vi "Fetch Waveform Measurement In Memory.vi"(6 "Measurement Number (0: Measurement 1)":i32(ring) items=["Measurement 1", "Measurement 2", "Measurement 3", "Measurement 4"], 7 "Destination Channel (1: Channel 2)":u16(ring)=1 items=["Channel 1", "Channel 2", "Channel 3", "Channel 4", "Math", "D0", "D1", "D2", "D3", "D4", "D5", "D6", "D7", "D8", "D9", "D10", "D11", "D12", "D13", "D14", "D15", "Reference 1", "Reference 2", "Reference 3", "Reference 4", "Amplitude", "Frequency", "Phase"], 8 "error in (no error)":errorcluster, 9 "Measurement Function (21: Period)":i32(ring)=21 items=["Amplitude", "Area", "Burst Width", "Cycle Area", "Voltage Mean (cycle)", "Voltage RMS (cycle)", "Delay", "Fall Time", "Frequency", "Voltage High", "Voltage Low", "Voltage Max", "Voltage Mean", "Voltage Min", "Negative Duty Cycle", "Negative Edges Count", "Negative Overshoot", "Negative Pulses Count", "Negative Pulse Width", "Positive Duty Cycle", "Positive Edges Count", "Period", "Phase", "Vpp", "Positive Overshoot", "Positive Pulses Count", "Positive Pulse Width", "Rise Time", "Voltage RMS", "Total Overshoot", "Histogram Hits", "Histogram Median", "Histogram Peak Hits", "Histogram Sigma 1", "Histogram Sigma 2", "Histogram Sigma 3", "Standard Deviation", "Waveform Count"], 10 "Channel (0: Channel 1)":u16(ring) items=["Channel 1", "Channel 2", "Channel 3", "Channel 4", "Math", "D0", "D1", "D2", "D3", "D4", "D5", "D6", "D7", "D8", "D9", "D10", "D11", "D12", "D13", "D14", "D15", "Reference 1", "Reference 2", "Reference 3", "Reference 4", "Amplitude", "Frequency", "Phase"], 11 "VISA resource name":refnum<visa-resource-name>) -> (0 "error out":errorcluster, 2 "Measurement Value":dbl, 3 "VISA resource name out":refnum<visa-resource-name>)   [LabVIEW 2017, in "Scope.lvlib" / "Tektronix DPO MSO 2000 4000 Series.lvlib"]
doc: "This VI fetches the displayed measurement value which is specified by the <B>Measurement Number</B>. \n\nFirstly, initiates an acquisition on the channel that you specify in the <B>Channel</B> control. After the acquisition completes, the Fetch Displayed Waveform Measurement VI performs displayed waveform measurement on the channel you specify and returns a measurement value. You can specify a measurement type, such as rise time, frequency, and voltage peak-to-peak, with this VI. Use the Fetch Displayed Waveform Measurement VI separately for any other waveform measurement on a channel without initiating another acquisition.\n\n<B>Notes:</B>\n\nThe <B>Fetch Waveform Measurement</B> VI returns the immediate measurement (which is what is typically done) while this VI returns the specified displayed measurement."
uses:
  Tektronix DPO MSO 2000 4000 Series.lvlib
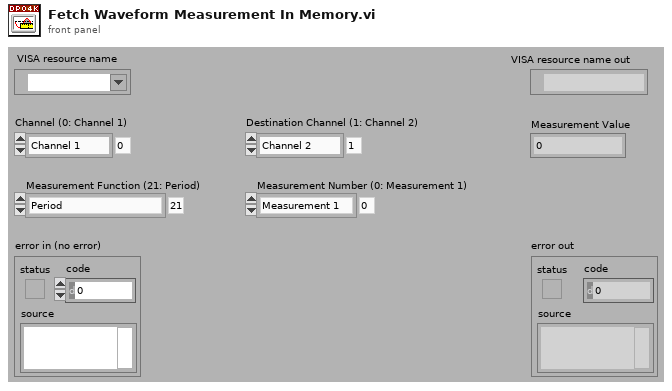
[diagram p1: front panel]
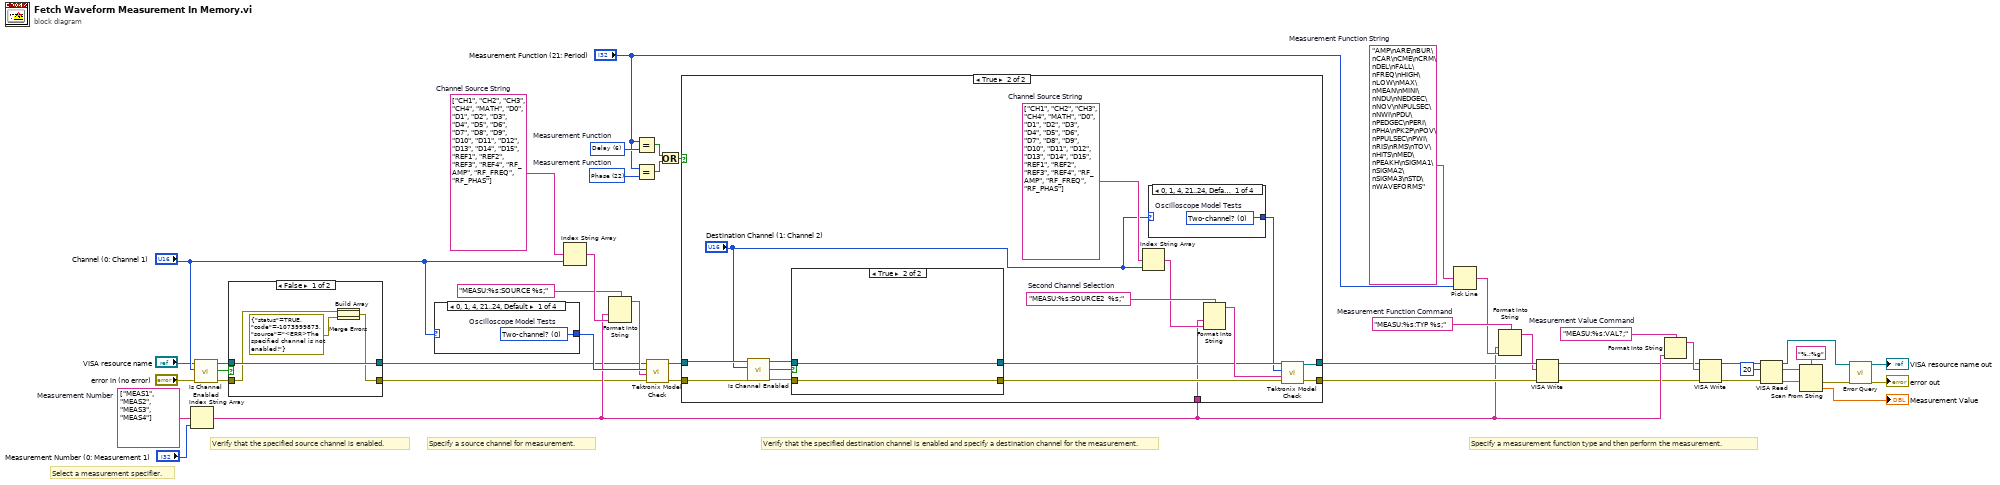
[diagram p0: block diagram]
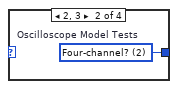
[diagram p3: hidden frame]
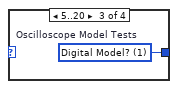
[diagram p4: hidden frame]
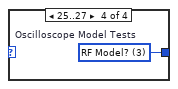
[diagram p5: hidden frame]
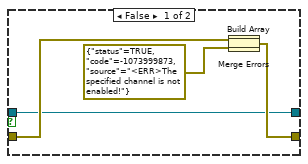
[diagram p6: hidden frame]
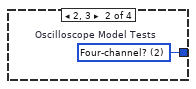
[diagram p7: hidden frame]
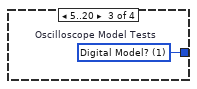
[diagram p8: hidden frame]
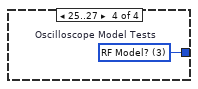
[diagram p9: hidden frame]
diagram:
  w11 = string[] ["MEAS1", "MEAS2", "MEAS3", "MEAS4"]  # Measurement Number
  w13 = "MEASU:%s:VAL?;"  # Measurement Value Command
  w28 = 22 items=["Amplitude", "Area", "Burst Width", "Cycle Area", "Voltage Mean (cycle)", "Voltage RMS (cycle)", "Delay", "Fall Time", "Frequency", "Voltage High", "Voltage Low", "Voltage Max", "Voltage Mean", "Voltage Min", "Negative Duty Cycle", "Negative Edges Count", "Negative Overshoot", "Negative Pulses Count", "Negative Pulse Width", "Positive Duty Cycle", "Positive Edges Count", "Period", "Phase", "Vpp", "Positive Overshoot", "Positive Pulses Count", "Positive Pulse Width", "Rise Time", "Voltage RMS"]  # Measurement Function
  w29 = 6 items=["Amplitude", "Area", "Burst Width", "Cycle Area", "Voltage Mean (cycle)", "Voltage RMS (cycle)", "Delay", "Fall Time", "Frequency", "Voltage High", "Voltage Low", "Voltage Max", "Voltage Mean", "Voltage Min", "Negative Duty Cycle", "Negative Edges Count", "Negative Overshoot", "Negative Pulses Count", "Negative Pulse Width", "Positive Duty Cycle", "Positive Edges Count", "Period", "Phase", "Vpp", "Positive Overshoot", "Positive Pulses Count", "Positive Pulse Width", "Rise Time", "Voltage RMS"]  # Measurement Function
  w37 = string[] ["CH1", "CH2", "CH3", "CH4", "MATH", "D0", "D1", "D2", "D3", "D4", "D5", "D6", "D7", "D8", "D9", "D10", "D11", "D12", "D13", "D14", "D15", "REF1", "REF2", "REF3", "REF4", "RF_AMP", "RF_FREQ", "RF_PHAS"]  # Channel Source String
  w44 = "MEASU:%s:TYP %s;"  # Measurement Function Command
  w45 = "AMP\nARE\nBUR\nCAR\nCME\nCRM\nDEL\nFALL\nFREQ\nHIGH\nLOW\nMAX\nMEAN\nMINI\nNDU\nNEDGEC\nNOV\nNPULSEC\nNWI\nPDU\nPEDGEC\nPERI\nPHA\nPK2P\nPOV\nPPULSEC\nPWI\nRIS\nRMS\nTOV\nHITS\nMED\nPEAKH\nSIGMA1\nSIGMA2\nSIGMA3\nSTD\nWAVEFORMS"  # Measurement Function String
  # "Select a measurement specifier."
  # "Specify a measurement function type and then perform the measurement."
  # "Specify a source channel for measurement."
  # "Verify that the specified destination channel is enabled and specify a destination channel for the measurement."
  # "Verify that the specified source channel is enabled."
  n1 = Index String Array(1:"Measurement Number (0: Measurement 1)", 2:w11) -> (0:w9:string)  [unwired: 1 in]
  n2 = call "Is Channel Enabled.vi"("error in (no error)"="error in (no error)", "Channel (0: Channel 1)"="Channel (0: Channel 1)", "VISA resource name"="VISA resource name") -> ("error out"=w40:errorcluster, "Enabled"=w41:bool, "VISA resource name out"=w39:refnum<visa-resource-name>)  [unwired: 6 in]
  n3 = case shown="False" w41 {
    tunnel: w40 -> [w48 w51]
    tunnel: w39 -> [w49 w52]
    tunnel: [w49 w52] -> w4
    tunnel: [w47 w51] -> w3
    frame False {
      n4 = Build Array(w48, errorcluster {"status"=TRUE, "code"=-1073999873, "source"="<ERR>The specified channel is not enabled!"} ("error out")) -> (w46:errorcluster[])
      n5 = Merge Errors(w46) -> (w47:errorcluster)
    }
    frame True {
    }
  }
  n6 = case shown="0, 1, 4, 21..24, Default" "Channel (0: Channel 1)" {
    tunnel: [w53 w54 w55 w56] -> w38
    frame 0, 1, 4, 21..24, Default {
      w53 = u16 0 items=["Two-channel?", "Digital Model?", "Four-channel?", "RF Model?"]  # Oscilloscope Model Tests
    }
    frame 2, 3 {
      w54 = u16 2 items=["Two-channel?", "Digital Model?", "Four-channel?", "RF Model?"]  # Oscilloscope Model Tests
    }
    frame 5..20 {
      w55 = u16 1 items=["Two-channel?", "Digital Model?", "Four-channel?", "RF Model?"]  # Oscilloscope Model Tests
    }
    frame 25..27 {
      w56 = u16 3 items=["Two-channel?", "Digital Model?", "Four-channel?", "RF Model?"]  # Oscilloscope Model Tests
    }
  }
  n7 = Index String Array(1:"Channel (0: Channel 1)", 2:w37) -> (0:w35:string)  [unwired: 1 in]
  n8 = Format Into String(format string="MEASU:%s:SOURCE %s;", w9, w35) -> (resulting string=w33:string)  [unwired: 2 in, 1 out]
  n9 = Equal?(x="Measurement Function (21: Period)", y=w29) -> (x = y?=w30:bool)
  n10 = Equal?(x="Measurement Function (21: Period)", y=w28) -> (x = y?=w31:bool)
  n11 = call "Tektronix Model Check.vi"("error in (no error)"=w3, "Command String"=w33, "Oscilloscope Model Tests (3: RF Model?)"=w38, "VISA resource name"=w4) -> ("error out"=w7:errorcluster, "VISA resource name out"=w8:refnum<visa-resource-name>)  [unwired: 6 in]
  n12 = Or(x=w30, y=w31) -> (x .or. y?=w27:bool)
  n13 = case shown="True" w27 {
    tunnel: w8 -> [w58 w67]
    tunnel: w7 -> [w57 w66]
    tunnel: [w58 w65] -> w25
    tunnel: [w57 w64] -> w24
    tunnel: w9 -> [_ w61]
    frame False {
    }
    frame True {
      w71 = string[] ["CH1", "CH2", "CH3", "CH4", "MATH", "D0", "D1", "D2", "D3", "D4", "D5", "D6", "D7", "D8", "D9", "D10", "D11", "D12", "D13", "D14", "D15", "REF1", "REF2", "REF3", "REF4", "RF_AMP", "RF_FREQ", "RF_PHAS"]  # Channel Source String
      w63 = "MEASU:%s:SOURCE2  %s;"  # Second Channel Selection
      n14 = call "Is Channel Enabled.vi"("error in (no error)"=w66, "Channel (0: Channel 1)"="Destination Channel (1: Channel 2)", "VISA resource name"=w67) -> ("error out"=w70:errorcluster, "Enabled"=w68:bool, "VISA resource name out"=w69:refnum<visa-resource-name>)  [unwired: 6 in]
      n15 = case shown="True" w68 {
        tunnel: w69 -> [w80 w85]
        tunnel: w70 -> [w82 w84]
        tunnel: [w80 w85] -> w72
        tunnel: [w81 w84] -> w73
        frame False {
          n16 = Build Array(w82, errorcluster {"status"=TRUE, "code"=-1073999873, "source"="<ERR>The specified channel is not enabled!"} ("error out")) -> (w79:errorcluster[])
          n17 = Merge Errors(w79) -> (w81:errorcluster)
        }
        frame True {
        }
      }
      n18 = Index String Array(1:"Destination Channel (1: Channel 2)", 2:w71) -> (0:w62:string)  [unwired: 1 in]
      n19 = case shown="0, 1, 4, 21..24, Default" "Destination Channel (1: Channel 2)" {
        tunnel: [w75 w76 w77 w78] -> w59
        frame 0, 1, 4, 21..24, Default {
          w75 = u16 0 items=["Two-channel?", "Digital Model?", "Four-channel?", "RF Model?"]  # Oscilloscope Model Tests
        }
        frame 2, 3 {
          w76 = u16 2 items=["Two-channel?", "Digital Model?", "Four-channel?", "RF Model?"]  # Oscilloscope Model Tests
        }
        frame 5..20 {
          w77 = u16 1 items=["Two-channel?", "Digital Model?", "Four-channel?", "RF Model?"]  # Oscilloscope Model Tests
        }
        frame 25..27 {
          w78 = u16 3 items=["Two-channel?", "Digital Model?", "Four-channel?", "RF Model?"]  # Oscilloscope Model Tests
        }
      }
      n20 = Format Into String(format string=w63, w61, w62) -> (resulting string=w74:string)  [unwired: 2 in, 1 out]
      n21 = call "Tektronix Model Check.vi"("error in (no error)"=w73, "Command String"=w74, "Oscilloscope Model Tests (3: RF Model?)"=w59, "VISA resource name"=w72) -> ("error out"=w64:errorcluster, "VISA resource name out"=w65:refnum<visa-resource-name>)  [unwired: 6 in]
    }
  }
  n22 = Pick Line(multi-line string=w45, line index="Measurement Function (21: Period)") -> (output string=w32:string)  [unwired: 1 in]
  n23 = Format Into String(format string=w44, w9, w32) -> (resulting string=w23:string)  [unwired: 2 in, 1 out]
  n24 = VISA Write(VISA resource name=w25, write buffer=w23, error in (no error)=w24) -> (VISA resource name out=w6:refnum<visa-resource-name>, error out=w5:errorcluster)  [unwired: 1 out]
  n25 = Format Into String(format string=w13, w9) -> (resulting string=w12:string)  [unwired: 2 in, 1 out]
  n26 = VISA Write(VISA resource name=w6, write buffer=w12, error in (no error)=w5) -> (VISA resource name out=w21:refnum<visa-resource-name>, error out=w20:errorcluster)  [unwired: 1 out]
  n27 = VISA Read(VISA resource name=w21, byte count=u32 20, error in (no error)=w20) -> (VISA resource name out=w17:refnum<visa-resource-name>, read buffer=w16:string, error out=w18:errorcluster)  [unwired: 1 out]
  n28 = Scan From String(format string="%.;%g", input string=w16, error in=w18) -> (error out=w15:errorcluster, output 1=→"Measurement Value":dbl)  [unwired: 2 in, 2 out]
  n29 = call "Error Query.vi"("error in (no error)"=w15, "VISA resource name"=w17) -> ("error out"=→"error out":errorcluster, "VISA resource name out"=→"VISA resource name out":refnum<visa-resource-name>)  [unwired: 6 in, 2 out]
